vi "AlliGator Decay Sum.vi"(1 "Output Plots":cluster{"t Array":dbl[], "I Array":dbl[]}[](array[cluster])) -> (0 "# Photons":dbl[](array[numeric]))   [LabVIEW 2021, in "AlliGator Fit Method Benchmark.lvlib"]
doc: "Computes the number of simulated photons in each decay (the other two plots are the fit and the residuals)."
uses:
  Tools/Fit Methods Comparison/AlliGator Fit Method Benchmark.lvlib
panel:
  # "see the AlliGator License on the block diagram (Ctrl+E or Window:Show Block Diagram)"
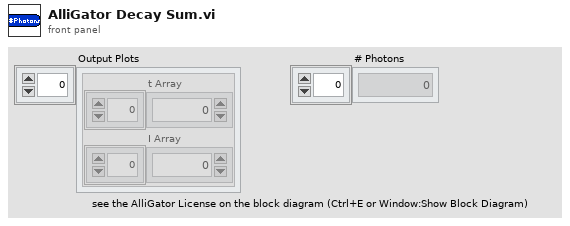
[diagram p1: front panel]
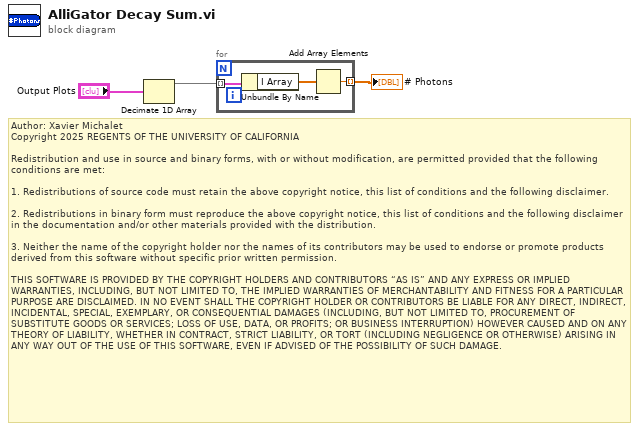
[diagram p0: block diagram]
diagram:
  # "Author: Xavier Michalet\nCopyright 2025 REGENTS OF THE UNIVERSITY OF CALIFORNIA\n\nRedistribution and use in source and binary forms, with or without modification, are permitted provided that the following conditions are met:\n\n1. Redistributions of source code must retain the above copyright notice, this list of conditions and the following disclaimer.\n\n2. Redistributions in binary form must reproduce the above copyright notice, this list of conditions and the following disclaimer in the documentation and/or other materials provided with the distribution.\n\n3. Neither the name of the copyright holder nor the names of its contributors may be used to endorse or promote products derived from this software without specific prior written permission.\n\nTHIS SOFTWARE IS PROVIDED BY THE COPYRIGHT HOLDERS AND CONTRIBUTORS “AS IS” AND ANY EXPRESS OR IMPLIED WARRANTIES, INCLUDING, BUT NOT LIMITED TO, THE IMPLIED WARRANTIES OF MERCHANTABILITY AND FITNESS FOR A PARTICULAR PURPOSE ARE DISCLAIMED. IN NO EVENT SHALL THE COPYRIGHT HOLDER OR CONTRIBUTORS BE LIABLE FOR ANY DIRECT, INDIRECT, INCIDENTAL, SPECIAL, EXEMPLARY, OR CONSEQUENTIAL DAMAGES (INCLUDING, BUT NOT LIMITED TO, PROCUREMENT OF SUBSTITUTE GOODS OR SERVICES; LOSS OF USE, DATA, OR PROFITS; OR BUSINESS INTERRUPTION) HOWEVER CAUSED AND ON ANY THEORY OF LIABILITY, WHETHER IN CONTRACT, STRICT LIABILITY, OR TORT (INCLUDING NEGLIGENCE OR OTHERWISE) ARISING IN ANY WAY OUT OF THE USE OF THIS SOFTWARE, EVEN IF ADVISED OF THE POSSIBILITY OF SUCH DAMAGE."
  n1 = Decimate 1D Array("Output Plots") -> (w1:cluster{"t Array":dbl[], "I Array":dbl[]}[])  [unwired: 2 out]
  n2 = for {
    tunnel: w1 -> [w6] mode=indexing
    tunnel: [w4] -> w2 mode=indexing
    n3 = Unbundle By Name(w6) -> ("I Array"=w5:dbl[])
    n4 = Add Array Elements(numeric array=w5) -> (sum=w4:dbl)
  }
  "# Photons" <- w2
